vi "Create OneOf Accessors.vi"(8 "error in (no error)":errorcluster, 10 "MessageElementMetadata":T1, 11 "Oneof Class Ref In":refnum<vi>) -> (0 "error out":errorcluster, 3 "Oneof Class Ref Out":refnum<vi>)   [LabVIEW 2019, in "gRPC Template Creation Utility.lvlib"]
uses:
  gRPC Template Creation Utility.lvlib
  TypeDefs/Message Element Type.ctl
  TypeDefs/Message Element Metadata (Scripting).ctl
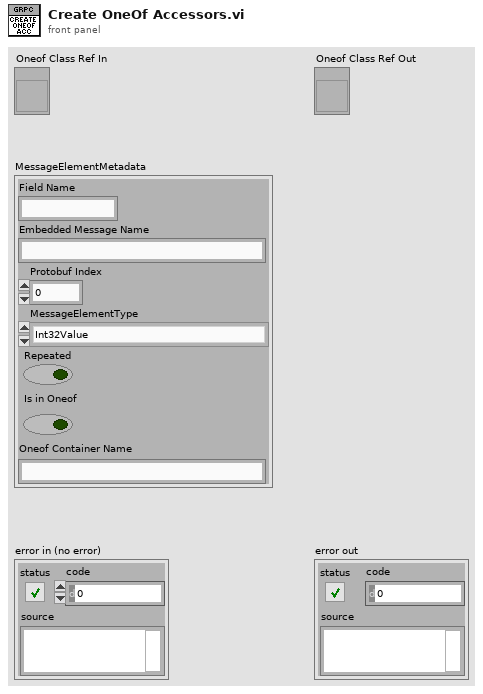
[diagram p1: front panel]
types:
  T1 = typedef "gRPC Template Creation Utility.lvlib/Message Element Metadata (Scripting).ctl" = cluster{"Field Name":string, "Embedded Message Name":string, "Protobuf Index":i32, "MessageElementType":T2, "Repeated":bool, "Is in Oneof":bool, "Oneof Container Name":string}
  T2 = typedef "gRPC Template Creation Utility.lvlib/Message Element Type.ctl" = enum32{"Int32Value", "FloatValue", "DoubleValue", "BoolValue", "StringValue", "MessageValue", "Int64Value", "UInt32Value", "UInt64Value", "EnumValue", "Bytes", "Fixed64", "Fixed32", "SFixed64", "SFixed32", "SInt64", "SInt32"}
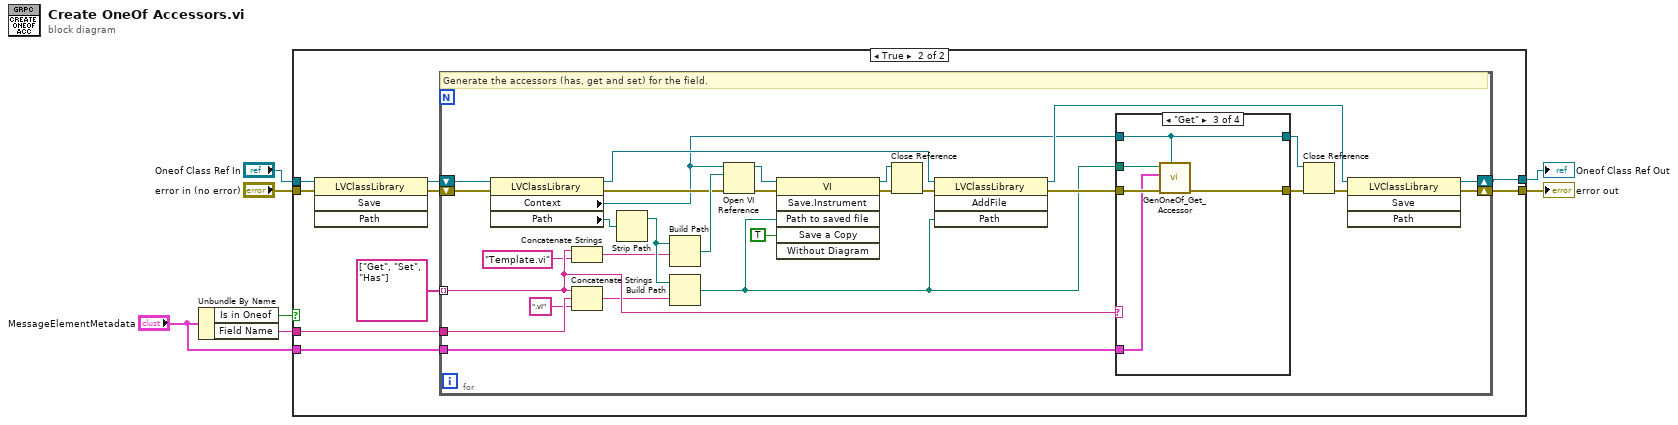
[diagram p0: block diagram]
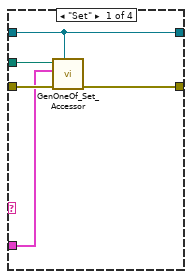
[diagram p3: hidden frame]
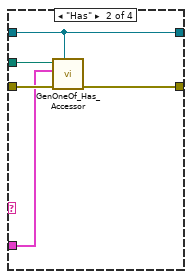
[diagram p4: hidden frame]
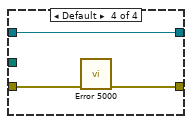
[diagram p5: hidden frame]
diagram:
  n1 = Unbundle By Name("MessageElementMetadata") -> ("Is in Oneof"=w5:bool, "Field Name"=w3:string)
  n2 = case shown="True" w5 {
    tunnel: "Oneof Class Ref In" -> [w8 w15]
    tunnel: w3 -> [_ w18]
    tunnel: [w9 w17] -> w4
    tunnel: "error in (no error)" -> [w9 w14]
    tunnel: [w8 w11] -> w2
    tunnel: "MessageElementMetadata" -> [_ w10]
    frame False {
    }
    frame True {
      n3 = invoke class="LVClassLibrary" method="Save"(reference=w15, error in=w14) -> (reference out=w12:refnum<vi>, error out=w13:errorcluster)  [unwired: 2 in, 2 out]
      n4 = for {
        tunnel: w18 -> [w46]
        shift-right: [w29] -> w17
        shift-left: w13 -> [w28]
        tunnel: string[] ["Get", "Set", "Has"] -> [w45] mode=indexing
        shift-right: [w26] -> w11
        shift-left: w12 -> [w47]
        tunnel: w10 -> [w22]
        # "Generate the accessors (has, get and set) for the field."
        n5 = property class="LVClassLibrary"(reference=w47, error in=w28) -> (reference out=w24:refnum<vi>, error out=w27:errorcluster, "Context"=w23:refnum<vi>, "Path"=w25:path)
        n6 = Concatenate Strings(w45, "Template.vi" ("Item Name")) -> (w39:string)
        n7 = Concatenate Strings(w45, w46, ".vi" ("string")) -> (w42:string)
        n8 = Strip Path(path=w25) -> (stripped path=w43:path)  [unwired: 1 out]
        n9 = Build Path(base path=w43, name or relative path=w39) -> (appended path=w36:path)
        n10 = Build Path(base path=w43, name or relative path=w42) -> (appended path=w37:path)
        n11 = Open VI Reference(application reference (local)=w23, vi path=w36, error in (no error)=w27) -> (vi reference=w34:refnum<vi>, error out=w35:errorcluster)  [unwired: 3 in]
        n12 = invoke class="VI" method="Save.Instrument"(reference=w34, error in=w35, "Path to saved file"=w37, "Save a Copy"=TRUE) -> (reference out=w31:refnum<vi>, error out=w32:errorcluster)  [unwired: 2 in, 4 out]
        n13 = Close Reference(reference=w31, error in (no error)=w32) -> (error out=w41:errorcluster)
        n14 = invoke class="LVClassLibrary" method="AddFile"(reference=w24, error in=w41, "Path"=w37) -> (reference out=w30:refnum<vi>, error out=w38:errorcluster)  [unwired: 1 in, 2 out]
        n15 = case shown="\"Get\"" w45 {
          tunnel: w38 -> [w52 w57 w62 w65]
          tunnel: w37 -> [w51 w56 w61 _]
          tunnel: [w50 w55 w60 w64] -> w21
          tunnel: w23 -> [w48 w53 w58 w63]
          tunnel: w22 -> [w49 w54 w59 _]
          tunnel: [w48 w53 w58 w63] -> w19
          frame "Set" {
            # "Edit the VI"
            n16 = call "GenOneOf_Set_Accessor.vi"("application reference"=w48, "error in (no error)"=w52, "message element metadata"=w49, "path"=w51) -> ("error out"=w50:errorcluster)  [unwired: 7 in]
          }
          frame "Has" {
            # "Edit the VI"
            n17 = call "GenOneOf_Has_Accessor.vi"("application reference"=w53, "error in (no error)"=w57, "message element metadata"=w54, "path"=w56) -> ("error out"=w55:errorcluster)  [unwired: 7 in]
          }
          frame "Get" {
            # "Edit the VI"
            n18 = call "GenOneOf_Get_Accessor.vi"("application reference"=w58, "error in (no error)"=w62, "message element metadata"=w59, "path"=w61) -> ("error out"=w60:errorcluster)  [unwired: 7 in]
          }
          frame Default {
            n19 = call "Error 5000.vi"("error in (no error)"=w65) -> ("error out"=w64:errorcluster)  [unwired: 10 in]
          }
        }
        n20 = Close Reference(reference=w19, error in (no error)=w21) -> (error out=w20:errorcluster)
        n21 = invoke class="LVClassLibrary" method="Save"(reference=w30, error in=w20) -> (reference out=w26:refnum<vi>, error out=w29:errorcluster)  [unwired: 2 in, 2 out]
      }
    }
  }
  "error out" <- w4
  "Oneof Class Ref Out" <- w2
